vi "Generate Context Help.vi"(8 "Help Information":T1, 9 "Device Name":string, 10 "Property Bundle":cluster{"Name":string, "Value":variant}[](array[cluster]), 11 "vi ref":T2) -> (2 "Dynamic Text Separator":string, 3 "Dynamic Text":string)   [LabVIEW 2021]
uses:
  <vilib>/myRIO/Common/Express VI Framework/typedefs/Config Pane Conn Pane Refnum.ctl
  <vilib>/myRIO/Common/Express VI Framework/vis/myRIOXB Global.vi
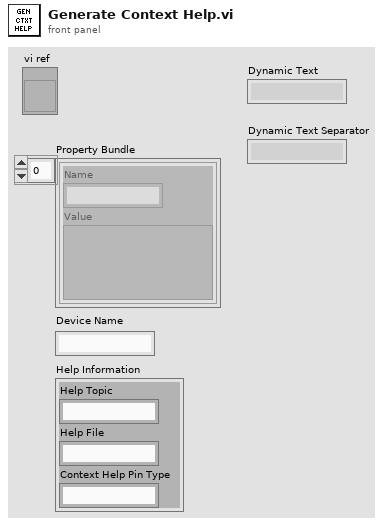
[diagram p1: front panel]
types:
  T1 = cluster{"Help Topic":string, "Help File":string, "Context Help Pin Type":string}
  T2 = typedef "Config Pane Conn Pane Refnum.ctl" = refnum<vi>
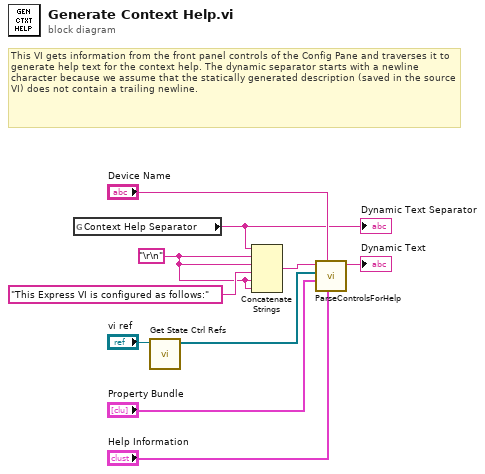
[diagram p0: block diagram]
diagram:
  w2 = "\r\n"
  # "This VI gets information from the front panel controls of the Config Pane and traverses it to generate help text for the context help. The dynamic separator starts with a newline character because we assume that the statically generated description (saved in the source VI) does not contain a trailing newline."
  n1 = global read "myRIOXB Global.vi" "Context Help Separator"() -> (w1:string)
  "Dynamic Text Separator" <- w1
  n2 = call <vilib>:"Get State Ctrl Refs.vi"("vi ref"="vi ref") -> ("All Controls[]"=w10:refnum<vi>[])  [unwired: 9 in, 1 out]
  n3 = Concatenate Strings(w1, w2, w2, "This Express VI is configured as follows:", w2, w2) -> (w8:string)
  n4 = call <vilib>:"ParseControlsForHelp.vi"("Help Information"="Help Information", "Device Name"="Device Name", "Property Bundle"="Property Bundle", "Control Refs"=w10, "String in"=w8) -> ("String out"=→"Dynamic Text":string)  [unwired: 5 in, 1 out]
